vi "PlaceBattleships.vi"(0 "object in":refnum<class "Map.lvclass">, 5 "error in (no error)":errorcluster) -> (14 "object out":refnum<class "Map.lvclass">, 16 "Failed":bool, 19 "error out":errorcluster)   [LabVIEW 2015, in "Map.lvclass"]
doc: "Randomly places all battleships on the map."
uses:
  Map.lvclass
  TypDefs/Coordinates.ctl
  Map.lvclass/Map.ctl
  Battleship_class/Battleship.lvclass
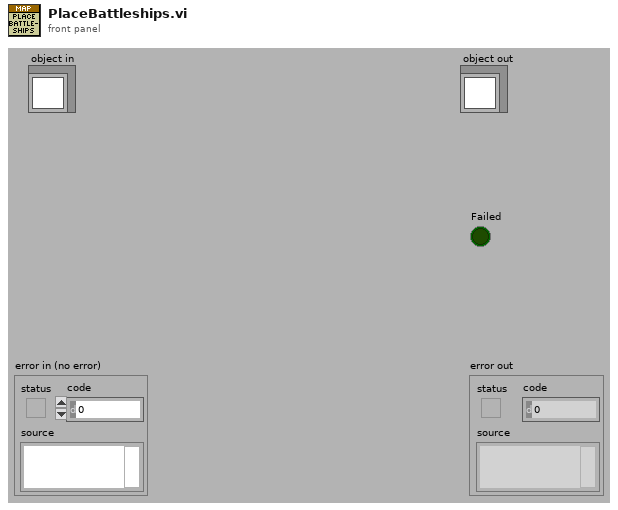
[diagram p1: front panel]
types:
  T1 = typedef "Coordinates.ctl" = cluster{"X":i32, "Y":i32}
  T2 = cluster{"State":string, "NrOfShips":i32, "ActiveShipIdx":i32, "Position":T1}
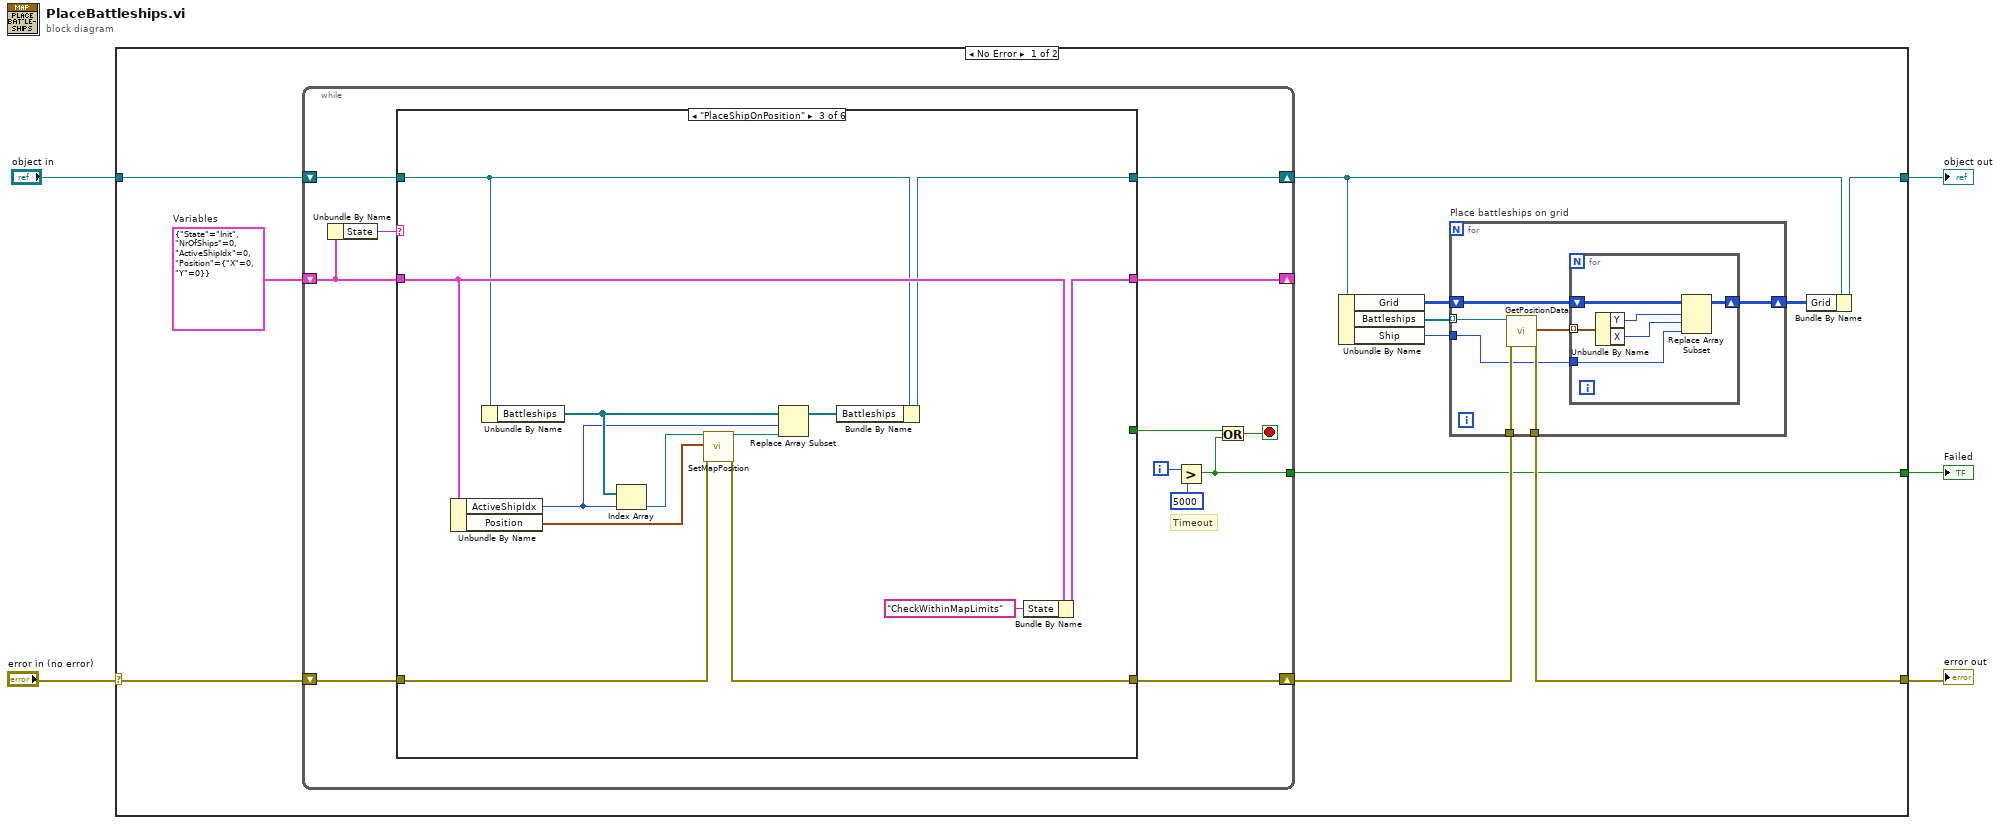
[diagram p0: block diagram]
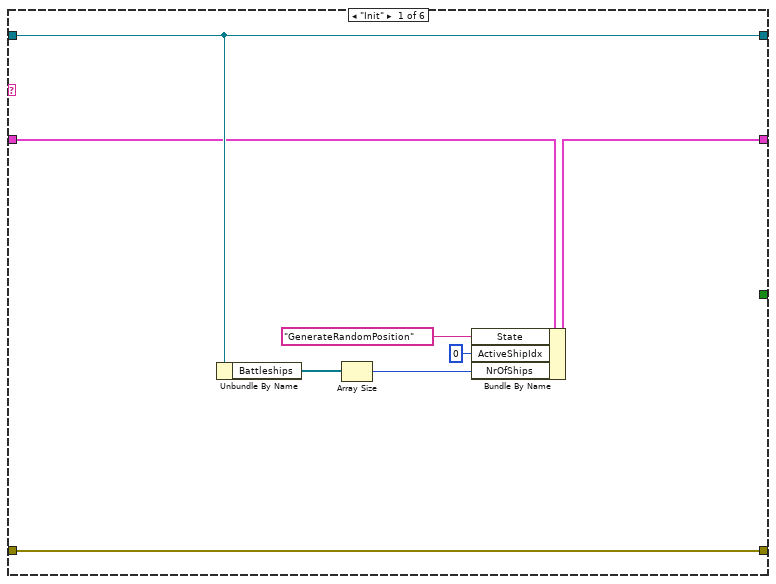
[diagram p2: hidden frame]
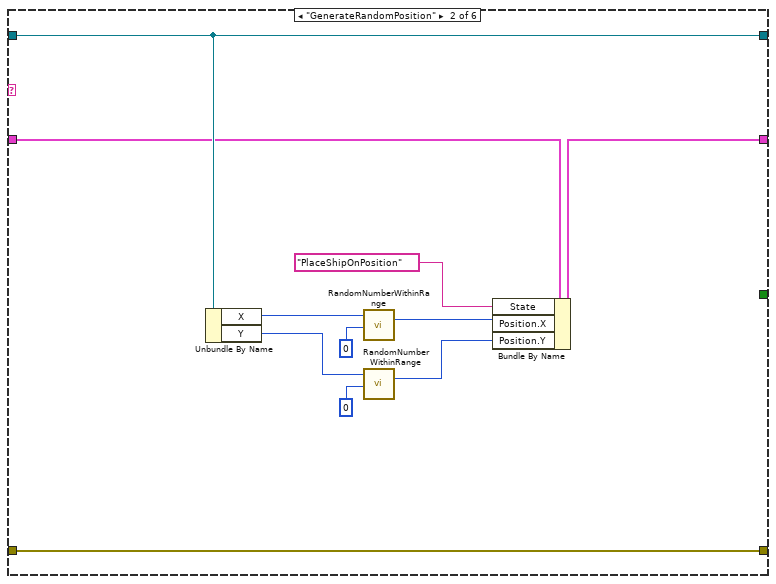
[diagram p3: hidden frame]
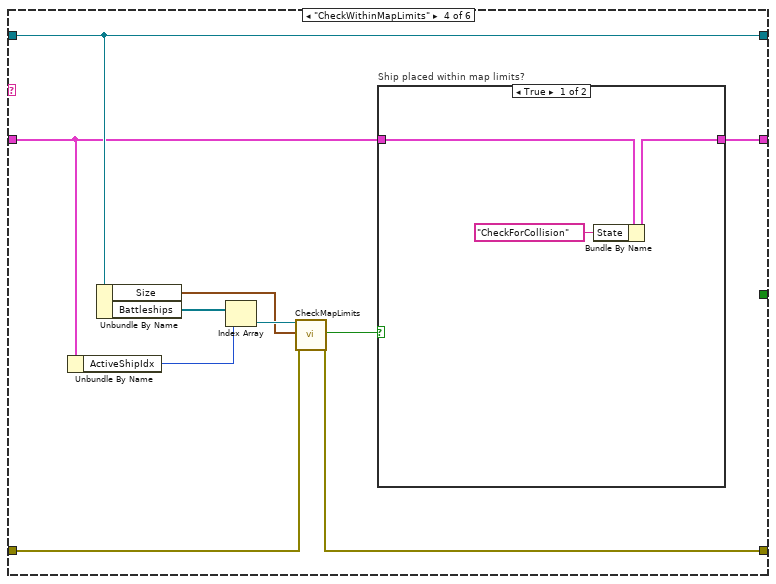
[diagram p4: hidden frame]
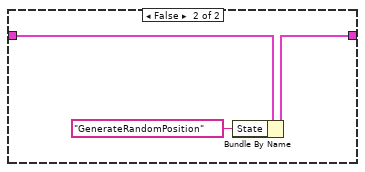
[diagram p5: hidden frame]
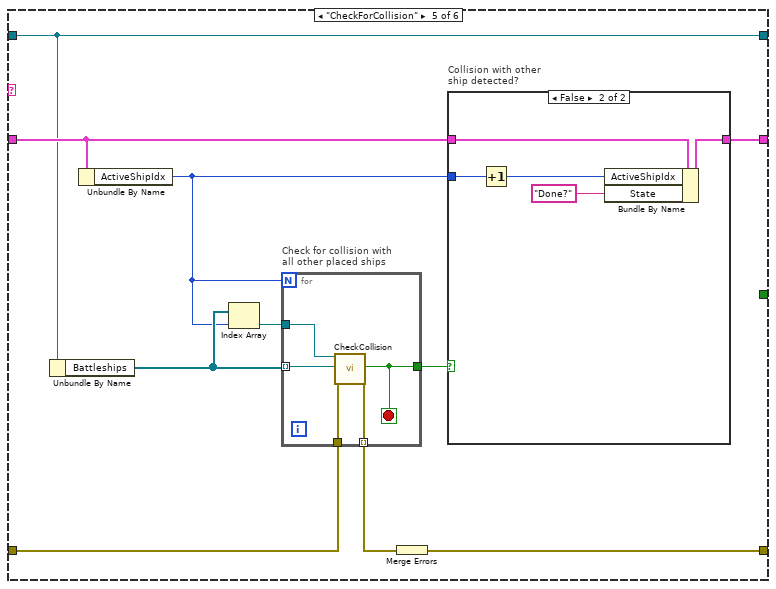
[diagram p6: hidden frame]
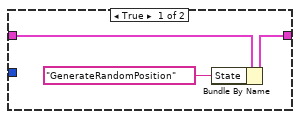
[diagram p7: hidden frame]
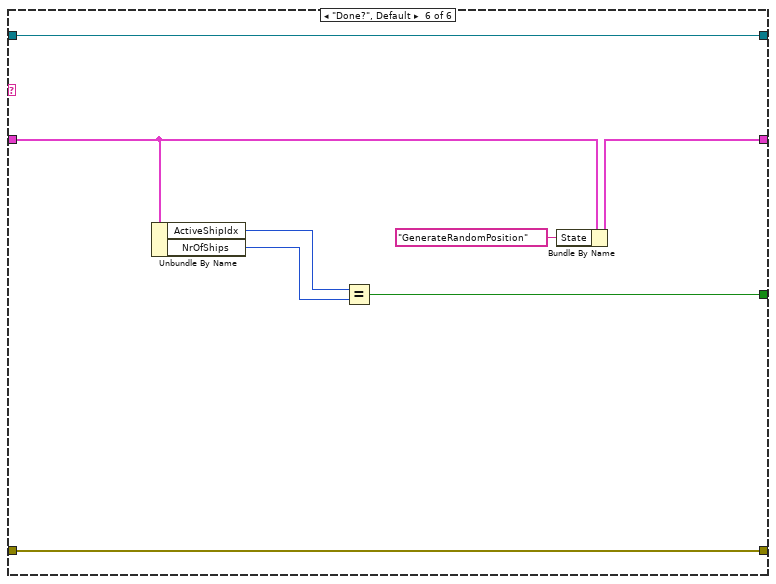
[diagram p8: hidden frame]
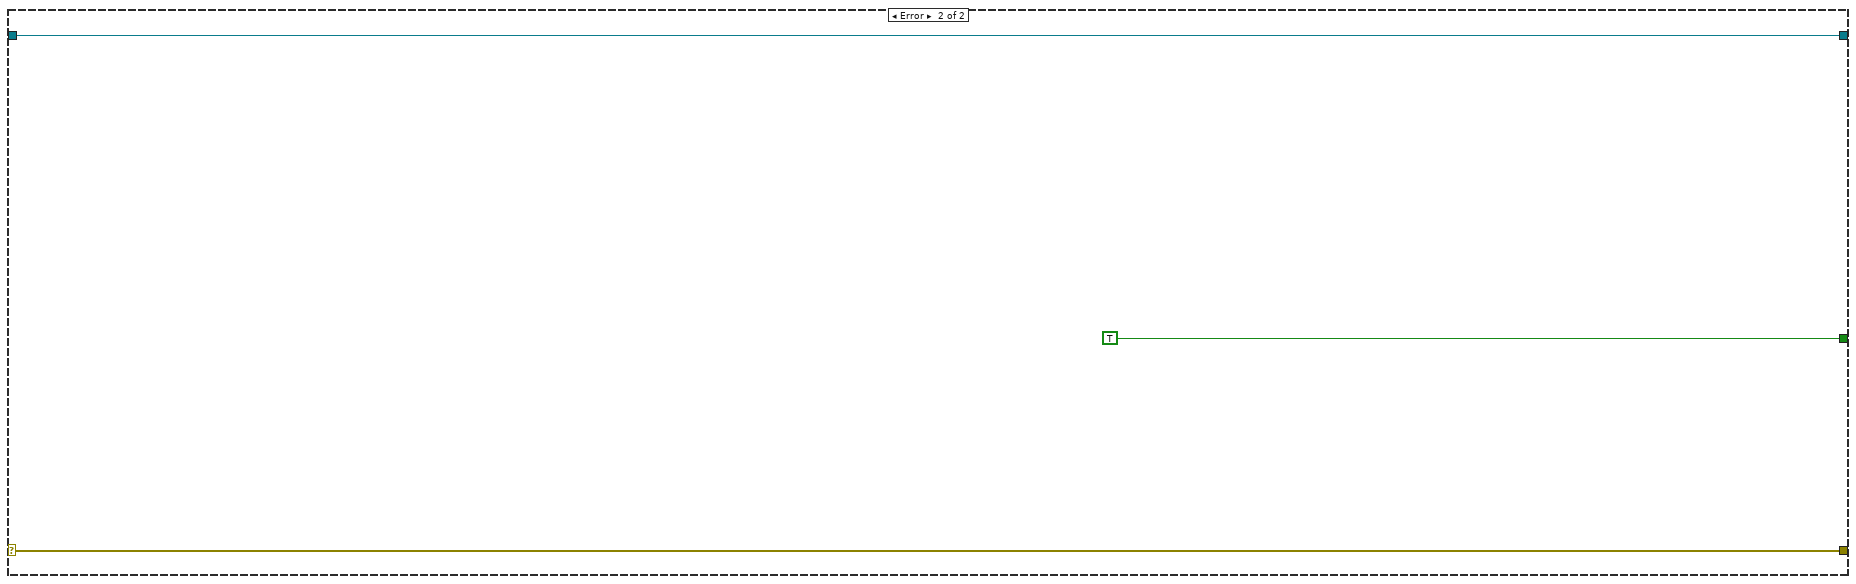
[diagram p9: hidden frame]
diagram:
  n1 = case shown="No Error" "error in (no error)" {
    selector: "error in (no error)" -> [w12 w124]
    tunnel: [w16 w124] -> w4
    tunnel: [w7 w123] -> w2
    tunnel: "object in" -> [w13 w123]
    tunnel: [w14 TRUE] -> w1
    frame No Error {
      w15 = T2 {"State"="Init", "NrOfShips"=0, "ActiveShipIdx"=0, "Position"={"X"=0, "Y"=0}}  # Variables
      n2 = while {
        shift-right: [w42] -> w11
        shift-left: w13 -> [w41]
        shift-right: [w36] -> _
        shift-left: w15 -> [w39]
        shift-right: [w38] -> w17
        shift-left: w12 -> [w37]
        tunnel: [w32] -> w14
        i -> [w35]
        stop <- w33 stop-if-true
        # "Timeout"
        n3 = Unbundle By Name(w39) -> ("State"=w40:string)
        n4 = case shown="\"PlaceShipOnPosition\"" w40 {
          tunnel: [w50 w61 w65 w84 w95 w121] -> w42
          tunnel: w41 -> [w50 w61 w70 w84 w95 w121]
          tunnel: w39 -> [w49 w56 w72 w76 w98 w119]
          tunnel: [w48 w54 w63 w77 w99 w115] -> w36
          tunnel: [w45 w55 w73 w78 w97 w120] -> w38
          tunnel: w37 -> [w45 w55 w74 w81 w96 w120]
          tunnel: [_ _ _ _ _ w118] -> w31
          frame "Init" {
            n5 = Unbundle By Name(w50) -> ("Battleships"=w47:refnum<class "Battleship.lvclass">[])
            n6 = Array Size(array=w47) -> (size(s)=w43:i32)
            n7 = Bundle By Name(cluster=w49, "State"="GenerateRandomPosition", "ActiveShipIdx"=0 ("ShipIndex"), "NrOfShips"=w43) -> (w48:T2)
          }
          frame "GenerateRandomPosition" {
            n8 = Unbundle By Name(w61) -> ("X"=w60:i32, "Y"=w59:i32)
            n9 = call "RandomNumberWithinRange.vi"("High"=w60, "Low"=0) -> ("Random Number"=w53:i32)  [unwired: 25 in]
            n10 = call "RandomNumberWithinRange.vi"("High"=w59, "Low"=0) -> ("Random Number"=w52:i32)  [unwired: 25 in]
            n11 = Bundle By Name(cluster=w56, "State"="PlaceShipOnPosition", "Position.X"=w53, "Position.Y"=w52) -> (w54:T2)
          }
          frame "PlaceShipOnPosition" {
            n12 = Unbundle By Name(w72) -> ("ActiveShipIdx"=w67:i32, "Position"=w71:T1)
            n13 = Unbundle By Name(w70) -> ("Battleships"=w68:refnum<class "Battleship.lvclass">[])
            n14 = Index Array(array=w68, index=w67) -> (element=w69:refnum<class "Battleship.lvclass">)
            n15 = call-dynamic "SetMapPosition.vi"("object in"=w69, "MapPosition"=w71, "error in (no error)"=w74) -> ("object out"=w66:refnum<class "Battleship.lvclass">, "error out"=w73:errorcluster)  [unwired: 15 in]
            n16 = Replace Array Subset(array=w68, new element=w66, index=w67) -> (w64:refnum<class "Battleship.lvclass">[])
            n17 = Bundle By Name(cluster=w70, "Battleships"=w64) -> (w65:refnum<class "Map.lvclass">)
            n18 = Bundle By Name(cluster=w72, "State"="CheckWithinMapLimits") -> (w63:T2)
          }
          frame "CheckWithinMapLimits" {
            n19 = Unbundle By Name(w76) -> ("ActiveShipIdx"=w79:i32)
            n20 = Unbundle By Name(w84) -> ("Size"=w82:T1, "Battleships"=w80:refnum<class "Battleship.lvclass">[])
            n21 = Index Array(array=w80, index=w79) -> (element=w83:refnum<class "Battleship.lvclass">)
            n22 = call-dynamic "CheckMapLimits.vi"("object in"=w83, "MapLimits"=w82, "error in (no error)"=w81) -> ("WithinMapLimits?"=w75:bool, "error out"=w78:errorcluster)  [unwired: 14 in, 1 out]
            n23 = case "Ship placed within map limits?" shown="True" w75 {
              tunnel: [w86 w89] -> w77
              tunnel: w76 -> [w87 w90]
              frame True {
                n24 = Bundle By Name(cluster=w87, "State"="CheckForCollision") -> (w86:T2)
              }
              frame False {
                n25 = Bundle By Name(cluster=w90, "State"="GenerateRandomPosition") -> (w89:T2)
              }
            }
          }
          frame "CheckForCollision" {
            n26 = Unbundle By Name(w95) -> ("Battleships"=w100:refnum<class "Battleship.lvclass">[])
            n27 = Unbundle By Name(w98) -> ("ActiveShipIdx"=w94:i32)
            n28 = Index Array(array=w100, index=w94) -> (element=w93:refnum<class "Battleship.lvclass">)
            n29 = for "Check for collision with\nall other placed ships" {
              N: w94 -> [_]
              tunnel: w93 -> [w113]
              tunnel: w100 -> [w112] mode=indexing
              tunnel: w96 -> [w111]
              tunnel: [w110] -> w92 mode=indexing
              tunnel: [w109] -> w91
              stop <- w109 stop-if-true
              n30 = call-dynamic "CheckCollision.vi"("object in"=w113, "Battleship"=w112, "error in (no error)"=w111) -> ("Collision?"=w109:bool, "error out"=w110:errorcluster)  [unwired: 14 in, 1 out]
            }
            n31 = Merge Errors(w92) -> (w97:errorcluster)
            n32 = case "Collision with other\nship detected?" shown="False" w91 {
              tunnel: [w102 w107] -> w99
              tunnel: w98 -> [w103 w108]
              tunnel: w94 -> [_ w106]
              frame True {
                n33 = Bundle By Name(cluster=w103, "State"="GenerateRandomPosition") -> (w102:T2)
              }
              frame False {
                n34 = Increment(x=w106) -> (x+1=w105:i32)
                n35 = Bundle By Name(cluster=w108, "ActiveShipIdx"=w105, "State"="Done?") -> (w107:T2)
              }
            }
          }
          frame "Done?", Default {
            n36 = Unbundle By Name(w119) -> ("ActiveShipIdx"=w117:i32, "NrOfShips"=w116:i32)
            n37 = Equal?(x=w117, y=w116) -> (x = y?=w118:bool)
            n38 = Bundle By Name(cluster=w119, "State"="GenerateRandomPosition") -> (w115:T2)
          }
        }
        n39 = Greater?(x=w35, y=5000 ("MaxIterations")) -> (0:w32:bool)
        n40 = Or(x=w31, y=w32) -> (x .or. y?=w33:bool)
      }
      n41 = Unbundle By Name(w11) -> ("Grid"=w10:u32[][], "Battleships"=w9:refnum<class "Battleship.lvclass">[], "Ship"=w8:u32)
      n42 = for "Place battleships on grid" {
        shift-right: [w21] -> w6
        shift-left: w10 -> [w22]
        tunnel: w9 -> [w20] mode=indexing
        tunnel: w8 -> [w18]
        tunnel: w17 -> [w24]
        tunnel: [w23] -> w16
        n43 = call-dynamic "GetPositionData.vi"("object in"=w20, "error in (no error)"=w24) -> ("MapPositions"=w19:T1[], "error out"=w23:errorcluster)  [unwired: 13 in, 3 out]
        n44 = for {
          tunnel: w19 -> [w28] mode=indexing
          shift-right: [w29] -> w21
          shift-left: w22 -> [w30]
          tunnel: w18 -> [w25]
          n45 = Unbundle By Name(w28) -> ("Y"=w27:i32, "X"=w26:i32)
          n46 = Replace Array Subset(array=w30, new element=w25, index (row)=w27, index (col)=w26) -> (w29:u32[][])
        }
      }
      n47 = Bundle By Name(cluster=w11, "Grid"=w6) -> (w7:refnum<class "Map.lvclass">)
    }
    frame Error {
    }
  }
  "error out" <- w4
  "object out" <- w2
  "Failed" <- w1
